vi "SlideLifetime.vi"(0 "rawdata":T1, 1 "window (photons)":u32, 2 "input range":cluster{"x0":dbl, "x1":dbl} {"x1" format="%.2f"; "x0" format="%.2f"}, 3 "channel count":i32, 4 "rebinning":i32, 5 "channel width (ns)":dbl format="%.2f", 6 "shift (photons)":u32) -> (7 "SlideLifetime":dbl[](array[numeric]) format="%.2f", 8 "SlideTime":dbl[](array[numeric]) format="%.2f")   [LabVIEW 2009]
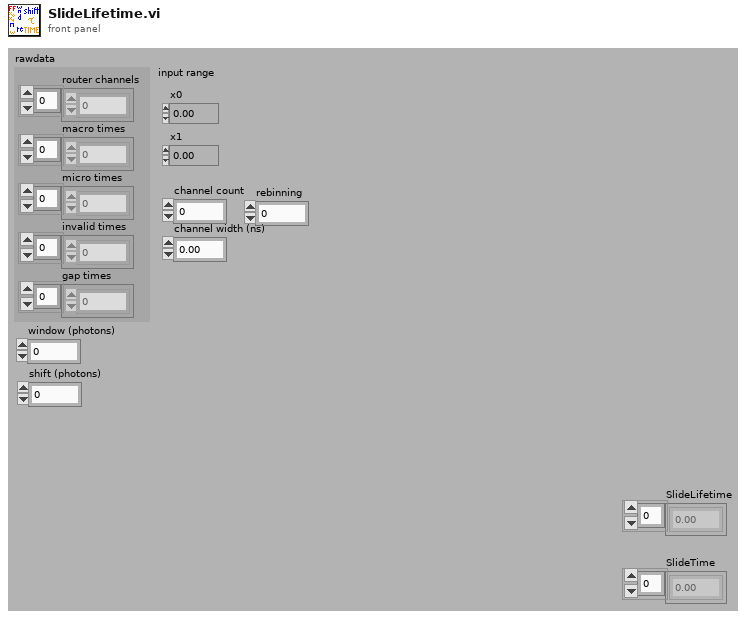
[diagram p1: front panel]
types:
  T1 = cluster{"router channels":u8[], "macro times":u32[], "micro times":u16[], "invalid times":u32[], "gap times":u32[]}
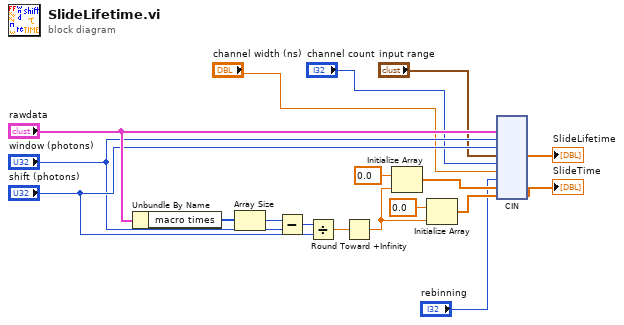
[diagram p0: block diagram]
diagram:
  n1 = Unbundle By Name("rawdata") -> ("macro times"=w15:u32[])
  n2 = Array Size(array=w15) -> (size(s)=w14:i32)
  n3 = Subtract(x=w14, y="window (photons)") -> (x-y=w13:u32)
  n4 = Divide(x=w13, y="shift (photons)") -> (x/y=w11:dbl)
  n5 = Round Toward +Infinity(x=w11) -> (ceil(x): smallest int >= x=w16:dbl)
  n6 = Initialize Array(0.0 ("element"), w16) -> (w7:dbl[])
  n7 = Initialize Array(0.0 ("element"), w16) -> (w9:dbl[])
  n8 = cin("rawdata", "window (photons)", "shift (photons)", "input range", "channel count", "channel width (ns)", "rebinning", w7, w9) -> (→"SlideLifetime":dbl[], →"SlideTime":dbl[])  [unwired: 7 in]
